vi "TCP Empty Buffer on Error.vi"(8 "Error In":errorcluster, 10 "timeout ms (1000)":i32=200, 11 "TCP Network Connection in":refnum<k5>) -> (0 "Error Out":errorcluster, 2 "String":string, 3 "TCP Network Connection out":refnum<k5>)   [LabVIEW 2020]
doc: "This software is licensed for use under the “MIT License\"\nCopyright (c) 2019 Scott Hannahs, sth@alum.mit.edu\n\nPermission is hereby granted, free of charge, to any person obtaining a copy of this software and associated documentation files (the \"Software\"), to deal in the Software without restriction, including without limitation the rights to use, copy, modify, merge, publish, distribute, sublicense, and/or sell copies of the Software, and to permit persons to whom the Software is furnished to do so, subject to the following conditions: The above copyright notice and this permission notice shall be included in all copies or substantial portions of the Software.\n\nTHE SOFTWARE IS PROVIDED \"AS IS\", WITHOUT WARRANTY OF ANY KIND, EXPRESS OR IMPLIED, INCLUDING BUT NOT LIMITED TO THE WARRANTIES OF MERCHANTABILITY, FITNESS FOR A PARTICULAR PURPOSE AND NONINFRINGEMENT. IN NO EVENT SHALL THE AUTHORS OR COPYRIGHT HOLDERS BE LIABLE FOR ANY CLAIM, DAMAGES OR OTHER LIABILITY, WHETHER IN AN ACTION OF CONTRACT, TORT OR OTHERWISE, ARISING FROM, OUT OF OR IN CONNECTION WITH THE SOFTWARE OR THE USE OR OTHER DEALINGS IN THE SOFTWARE."
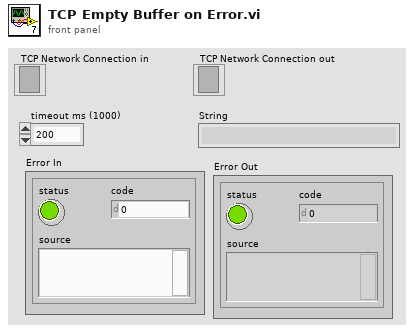
[diagram p1: front panel]
types:
  T1 = enum16{"Standard", "Buffered", "CRLF", "Immediate"}
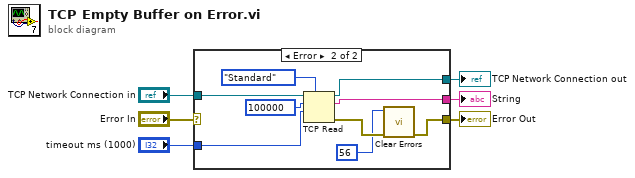
[diagram p0: block diagram]
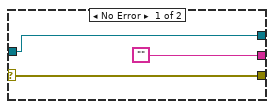
[diagram p2: hidden frame]
diagram:
  n1 = case shown="Error" "Error In" {
    selector: "Error In" -> [w7 _]
    tunnel: "timeout ms (1000)" -> [_ w18]
    tunnel: [w9 w15] -> w5
    tunnel: "TCP Network Connection in" -> [w9 w14]
    tunnel: [w7 w11] -> w3
    tunnel: ["" w12] -> w2
    frame No Error {
    }
    frame Error {
      n2 = TCP Read(connection ID=w14, bytes to read=100000, 7:T1."Standard" ("mode (standard)"), 9:w18) -> (connection ID out=w15:refnum<k5>, data out=w12:string, error out=w13:errorcluster)  [unwired: 1 in]
      n3 = call <vilib>:"Clear Errors.vi"("error in (no error)"=w13, "specific error code to clear (0: all)"=56) -> ("error out"=w11:errorcluster)  [unwired: 4 in, 1 out]
    }
  }
  "String" <- w2
  "TCP Network Connection out" <- w5
  "Error Out" <- w3
